vi "cRIO Module Info.vi"(8 "error in":errorcluster, 10 "Module":u16, 11 "Refnum in":refnum<k20>) -> (0 "error out":errorcluster, 2 "cRIO Module Info":T1 {"Serial Number" format="%.0x"; "Vendor and Module ID" format="%.0x"}, 3 "Refnum out":refnum<k20>)   [LabVIEW 2015, in "CRI.lvlib"]
uses:
  Perforce/Sales/projects/Components/CRI/trunk/source/lv2015/vi.lib/NI/CRI/CRI.lvlib
  Perforce/Sales/projects/Components/CRI/trunk/source/lv2015/vi.lib/NI/CRI/_subVIs/TypeDefs/cRIO Module Info.ctl
  <vilib>/Utility/error.llb/Error Cluster From Error Code.vi
  <vilib>/rvi/errors/niLvFpgaAdjustHostInterfaceError.vi
  <vilib>/rvi/interface/nirviReadWriteControl/nirviReadWriteControl.xnode
  <vilib>/ErrorRing/Error Ring.xnode
  NiFpgaLv.dll
  <vilib>/rvi/interface/Simulation/niFpgaSimulationCallBeginRW.vi
  Module.lvclass
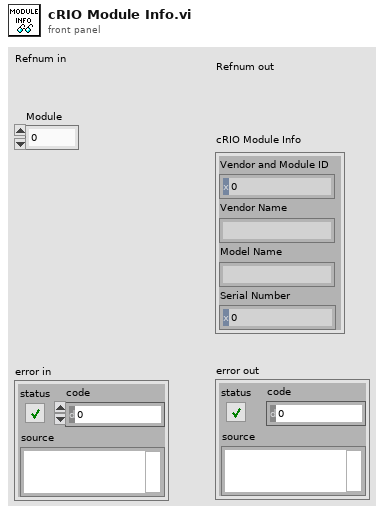
[diagram p1: front panel]
types:
  T1 = typedef "CRI.lvlib/cRIO Module Info.ctl" = cluster{"Vendor and Module ID":u32, "Vendor Name":string, "Model Name":string, "Serial Number":u32}
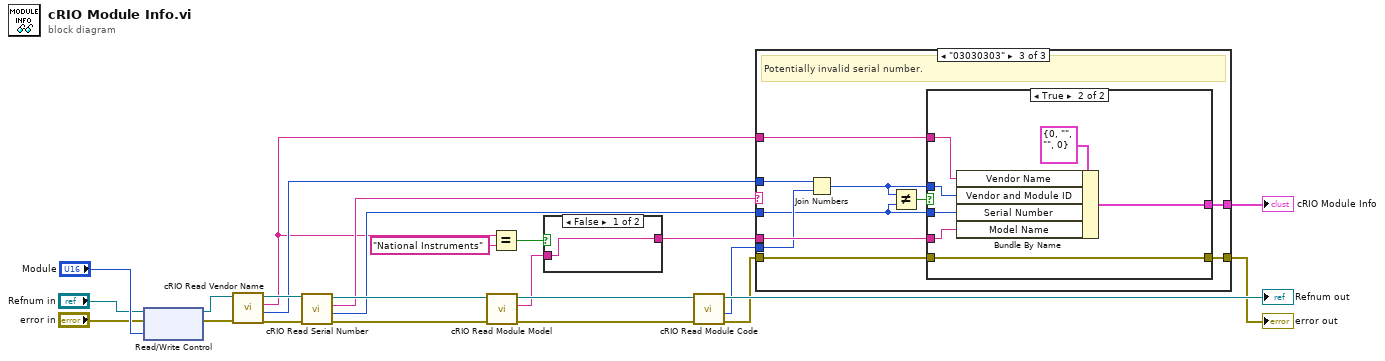
[diagram p0: block diagram]
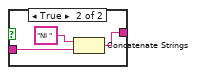
[diagram p2: hidden frame]
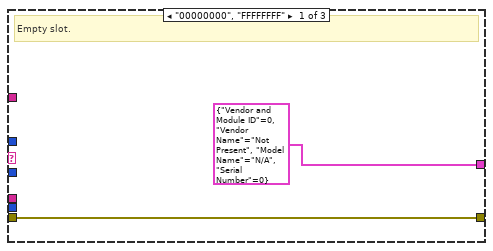
[diagram p3: hidden frame]
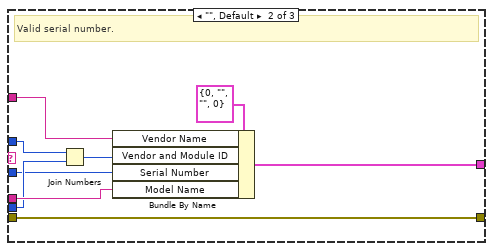
[diagram p4: hidden frame]
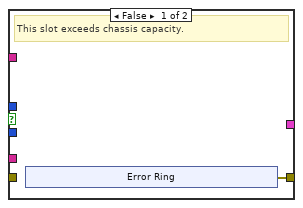
[diagram p5: hidden frame]
diagram:
  n1 = xnode "Read/Write Control"("FPGA VI Reference In"="Refnum in", "error in"="error in", "Module"="Module") -> ("FPGA VI Reference Out"=w18:refnum<k20>, "error out"=w19:errorcluster)
  n2 = call "cRIO Read Vendor Name.vi"("error in"=w19, "Refnum in"=w18) -> ("error out"=w21:errorcluster, "Vendor ID"=w11:u16, "Vendor Name"=w7:string, "Refnum out"=w22:refnum<k20>)  [unwired: 6 in]
  n3 = call "cRIO Read Serial Number.vi"("error in"=w21, "Refnum in"=w22) -> ("error out"=w24:errorcluster, "Serial Number"=w8:u32, "Serial Number String"=w15:string, "Refnum out"=w23:refnum<k20>)  [unwired: 6 in]
  n4 = call "cRIO Read Module Model.vi"("error in"=w24, "Refnum in"=w23) -> ("error out"=w14:errorcluster, "Module Model"=w4:string, "Refnum out"=w13:refnum<k20>)  [unwired: 7 in]
  n5 = Equal?(x=w7, y="National Instruments") -> (x = y?=w5:bool)
  n6 = case shown="False" w5 {
    tunnel: w4 -> [w25 w27]
    tunnel: [w25 w26] -> w3
    frame False {
    }
    frame True {
      n7 = Concatenate Strings("NI " ("string"), w27) -> (w26:string)
    }
  }
  n8 = call "cRIO Read Module Code.vi"("error in"=w14, "Refnum in"=w13) -> ("error out"=w2:errorcluster, "Module ID"=w9:u16, "Refnum out"=→"Refnum out":refnum<k20>)  [unwired: 6 in, 1 out]
  n9 = case shown="\"03030303\"" w15 {
    tunnel: w7 -> [_ w39 w49]
    tunnel: w3 -> [_ w38 w48]
    tunnel: [T1 {"Vendor and Module ID"=0, "Vendor Name"="Not Present", "Model Name"="N/A", "Serial Number"=0} ("cRIO Module Info") w37 w47] -> w10
    tunnel: w9 -> [_ w36 w46]
    tunnel: w11 -> [_ w35 w45]
    tunnel: w8 -> [_ w34 w40]
    tunnel: w2 -> [w29 w31 w43]
    tunnel: [w29 w31 w42] -> w1
    frame "00000000", "FFFFFFFF" {
      # "Empty slot."
    }
    frame "", Default {
      # "Valid serial number."
      n10 = Join Numbers(hi=w35, lo=w36) -> ((hi.lo)=w32:u32)
      n11 = Bundle By Name(cluster=T1 {"Vendor and Module ID"=0, "Vendor Name"="", "Model Name"="", "Serial Number"=0} ("cRIO Module Info"), "Vendor Name"=w39, "Vendor and Module ID"=w32, "Serial Number"=w34, "Model Name"=w38) -> (w37:T1)
    }
    frame "03030303" {
      # "Potentially invalid serial number."
      n12 = Join Numbers(hi=w45, lo=w46) -> ((hi.lo)=w41:u32)
      n13 = Not Equal?(x=w41, y=w40) -> (x != y?=w44:bool)
      n14 = case shown="True" w44 {
        tunnel: w49 -> [_ w61]
        tunnel: w48 -> [_ w60]
        tunnel: [_ w59] -> w47
        tunnel: w40 -> [_ w58]
        tunnel: w41 -> [_ w56]
        tunnel: w43 -> [_ w55]
        tunnel: [w50 w55] -> w42
        frame False {
          # "This slot exceeds chassis capacity."
          n15 = xnode "Error Ring"() -> ("error out"=w50:errorcluster)
        }
        frame True {
          n16 = Bundle By Name(cluster=T1 {"Vendor and Module ID"=0, "Vendor Name"="", "Model Name"="", "Serial Number"=0} ("cRIO Module Info"), "Vendor Name"=w61, "Vendor and Module ID"=w56, "Serial Number"=w58, "Model Name"=w60) -> (w59:T1)
        }
      }
    }
  }
  "error out" <- w1
  "cRIO Module Info" <- w10
